vi "Mecanum_Calc.vi"(8 "Max Speed":dbl=3600.0, 11 "Drive Command Inputs":T1) -> (0 "error out":errorcluster, 3 "Drive Outputs":T2)   [LabVIEW 2012]
panel:
  in  "Dividing Factor":dbl=2.5
  in  "Set PID":bool
  in  "P Left":dbl
  in  "I Left":dbl=0.01
  in  "D Left":dbl
  in  "P Right":dbl
  in  "I Right":dbl=0.01
  in  "D Right":dbl
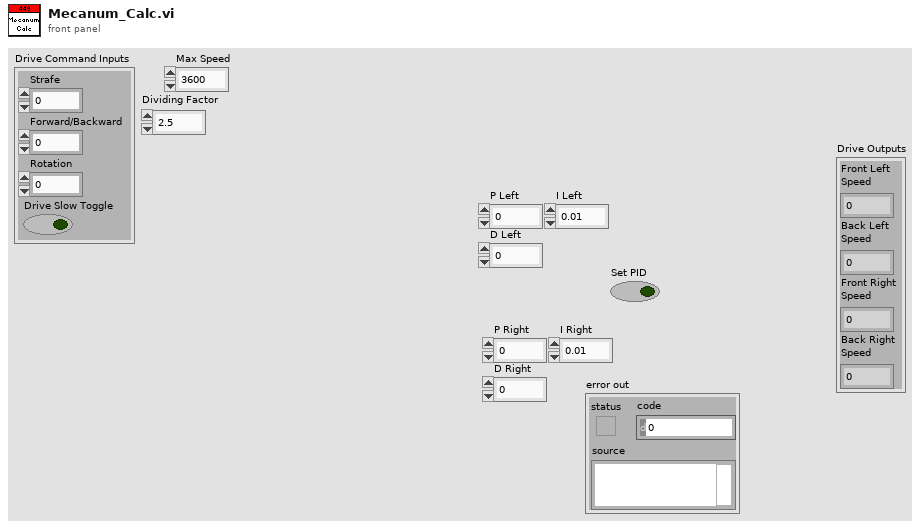
[diagram p1: front panel]
types:
  T1 = cluster{"Strafe":dbl, "Forward/Backward":dbl, "Rotation":dbl, "Drive Slow Toggle":bool}
  T2 = cluster{"Front Left\nSpeed":dbl, "Back Left\nSpeed":dbl, "Front Right\nSpeed":dbl, "Back Right\nSpeed":dbl}
  T3 = typedef "WPI_MotorControlDeviceRef.ctl" = cluster{"DeviceStatus":errorcluster, "Type":enum16{"PWM", "CAN"}, "PWM":cluster{"Digital Module":T4, "PWM Channel":T5, "DeadBand":T6}, "CAN":cluster{"Device Number":u8, "Control Mode":T7, "Semaphore":T8, "Max Vout":dbl}, "Invert":bool, "TransformRef":T9, "InvTransformRef":T9}
  T4 = typedef "FPGA_TypedefDigitalModule.ctl" = enum16{"Digital Module 1", "Digital Module 2"}
  T5 = typedef "FPGA_DIOPWMChannel.ctl" = enum8{"PWM 1", "PWM 2", "PWM 3", "PWM 4", "PWM 5", "PWM 6", "PWM 7", "PWM 8", "PWM 9", "PWM 10", "Invalid"}
  T6 = typedef "WPI_PWMDeadband.ctl" = cluster{"Name":string, "maxPositivePwm":i32, "minPositivePwm":i32, "centerPwm":i32, "maxNegativePwm":i32, "minNegativePwm":i32, "angularRange":u16}
  T7 = typedef "WPI_CANJaguar_ControlMode.ctl" = enum8{"Percent VBus", "Current", "Speed", "Position", "Voltage"}
  T8 = typedef "Semaphore RefNum" = refnum<k1>
  T9 = typedef "WPI_PWMTransform_ConPane.ctl" = refnum<vi>
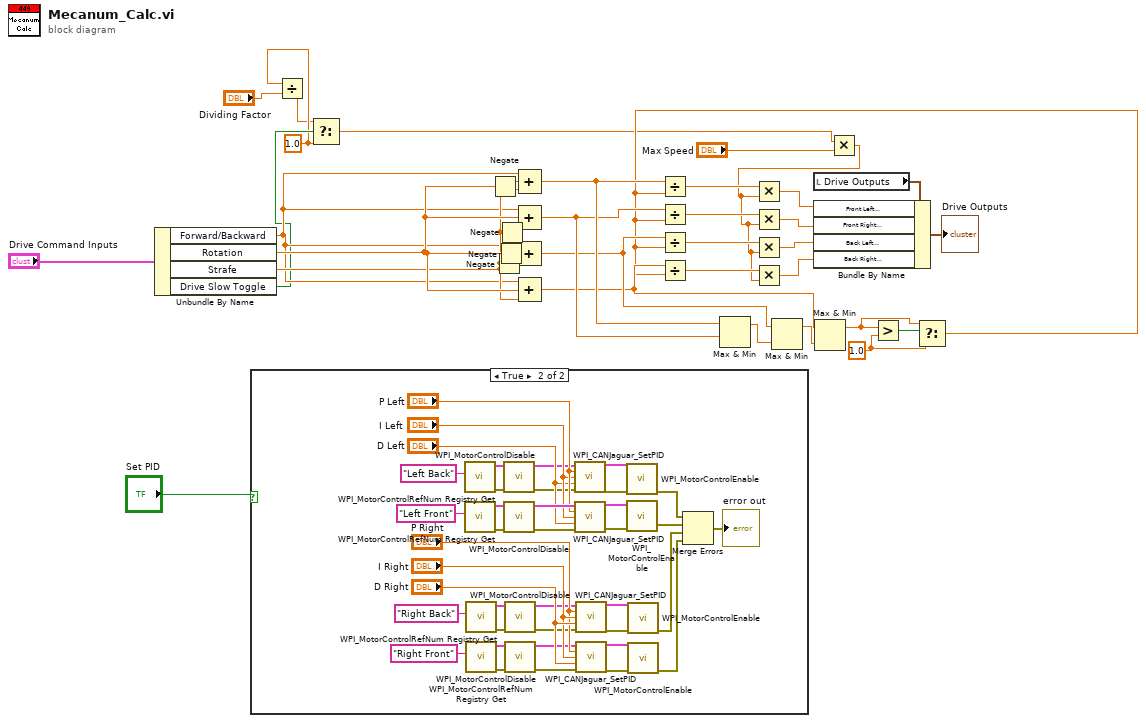
[diagram p0: block diagram]
diagram:
  w2 = 1.0 ("f")
  w17 = 1.0 ("y")
  n1 = Unbundle By Name("Drive Command Inputs") -> ("Forward/Backward"=w5:dbl, "Rotation"=w11:dbl, "Strafe"=w10:dbl, "Drive Slow Toggle"=w4:bool)
  n2 = case shown="True" "Set PID" {
    frame False {
    }
    frame True {
      n3 = call <vilib>:"WPI_MotorControlRefNum Registry Get.vi"("refnum name"="Left Back") -> ("error out"=w57:errorcluster, "MotorControlDevRef"=w56:T3)  [unwired: 9 in]
      n4 = call <vilib>:"WPI_MotorControlRefNum Registry Get.vi"("refnum name"="Left Front") -> ("error out"=w71:errorcluster, "MotorControlDevRef"=w72:T3)  [unwired: 9 in]
      n5 = call <vilib>:"WPI_MotorControlRefNum Registry Get.vi"("refnum name"="Right Back") -> ("error out"=w39:errorcluster, "MotorControlDevRef"=w40:T3)  [unwired: 9 in]
      n6 = call <vilib>:"WPI_MotorControlRefNum Registry Get.vi"("refnum name"="Right Front") -> ("error out"=w50:errorcluster, "MotorControlDevRef"=w49:T3)  [unwired: 9 in]
      n7 = call <vilib>:"WPI_MotorControlDisable.vi"("error in (no error)"=w57, "MotorControlDevRef"=w56) -> ("error out"=w54:errorcluster, "MotorControlDevRef"=w55:T3)  [unwired: 8 in]
      n8 = call <vilib>:"WPI_MotorControlDisable.vi"("error in (no error)"=w71, "MotorControlDevRef"=w72) -> ("error out"=w74:errorcluster, "MotorControlDevRef"=w73:T3)  [unwired: 8 in]
      n9 = call <vilib>:"WPI_MotorControlDisable.vi"("error in (no error)"=w39, "MotorControlDevRef"=w40) -> ("error out"=w42:errorcluster, "MotorControlDevRef"=w41:T3)  [unwired: 8 in]
      n10 = call <vilib>:"WPI_MotorControlDisable.vi"("error in (no error)"=w50, "MotorControlDevRef"=w49) -> ("error out"=w47:errorcluster, "MotorControlDevRef"=w48:T3)  [unwired: 8 in]
      n11 = call <vilib>:"WPI_CANJaguar_SetPID.vi"("CAN Jaguar Ref"=w55, "P"="P Left", "I"="I Left", "D"="D Left", "error in (no error)"=w54) -> ("CAN Jaguar Ref Out"=w53:T3, "error out"=w52:errorcluster)  [unwired: 9 in]
      n12 = call <vilib>:"WPI_CANJaguar_SetPID.vi"("CAN Jaguar Ref"=w73, "P"="P Left", "I"="I Left", "D"="D Left", "error in (no error)"=w74) -> ("CAN Jaguar Ref Out"=w75:T3, "error out"=w37:errorcluster)  [unwired: 9 in]
      n13 = call <vilib>:"WPI_CANJaguar_SetPID.vi"("CAN Jaguar Ref"=w41, "P"="P Right", "I"="I Right", "D"="D Right", "error in (no error)"=w42) -> ("CAN Jaguar Ref Out"=w43:T3, "error out"=w44:errorcluster)  [unwired: 9 in]
      n14 = call <vilib>:"WPI_CANJaguar_SetPID.vi"("CAN Jaguar Ref"=w48, "P"="P Right", "I"="I Right", "D"="D Right", "error in (no error)"=w47) -> ("CAN Jaguar Ref Out"=w46:T3, "error out"=w45:errorcluster)  [unwired: 9 in]
      n15 = call <vilib>:"WPI_MotorControlEnable.vi"("error in (no error)"=w52, "CAN Jaguar Ref"=w53) -> ("error out"=w69:errorcluster)  [unwired: 8 in, 1 out]
      n16 = call <vilib>:"WPI_MotorControlEnable.vi"("error in (no error)"=w37, "CAN Jaguar Ref"=w75) -> ("error out"=w68:errorcluster)  [unwired: 8 in, 1 out]
      n17 = call <vilib>:"WPI_MotorControlEnable.vi"("error in (no error)"=w44, "CAN Jaguar Ref"=w43) -> ("error out"=w67:errorcluster)  [unwired: 8 in, 1 out]
      n18 = call <vilib>:"WPI_MotorControlEnable.vi"("error in (no error)"=w45, "CAN Jaguar Ref"=w46) -> ("error out"=w66:errorcluster)  [unwired: 8 in, 1 out]
      n19 = Merge Errors(w69, w68, w67, w66) -> (→"error out":errorcluster)
    }
  }
  n20 = Divide(x=w2, y="Dividing Factor") -> (x/y=w1:dbl)
  n21 = Select(t=w1, s=w4, f=w2) -> (s? t:f=w14:dbl)
  n22 = Negate(x=w11) -> (-x=w6:dbl)
  n23 = Negate(x=w10) -> (-x=w8:dbl)
  n24 = Negate(x=w11) -> (-x=w9:dbl)
  n25 = Negate(x=w10) -> (-x=w7:dbl)
  n26 = Compound Arithmetic op=ADD(w5, w6, w10) -> (w25:dbl)
  n27 = Compound Arithmetic op=ADD(w5, w11, w7) -> (w24:dbl)
  n28 = Compound Arithmetic op=ADD(w5, w9, w8) -> (w23:dbl)
  n29 = Compound Arithmetic op=ADD(w5, w11, w10) -> (w21:dbl)
  n30 = Max & Min(x=w25, y=w24) -> (max(x,y)=w22:dbl)  [unwired: 1 out]
  n31 = Max & Min(x=w23, y=w22) -> (max(x,y)=w20:dbl)  [unwired: 1 out]
  n32 = local read "Drive Outputs"() -> (w35:T2)
  n33 = Max & Min(x=w21, y=w20) -> (max(x,y)=w18:dbl)  [unwired: 1 out]
  n34 = Multiply(x=w14, y="Max Speed") -> (x*y=w12:dbl)
  n35 = Greater?(x=w18, y=w17) -> (0:w19:bool)
  n36 = Select(t=w18, s=w19, f=w17) -> (s? t:f=w16:dbl)
  n37 = Divide(x=w25, y=w16) -> (x/y=w26:dbl)
  n38 = Divide(x=w24, y=w16) -> (x/y=w31:dbl)
  n39 = Divide(x=w23, y=w16) -> (x/y=w34:dbl)
  n40 = Divide(x=w21, y=w16) -> (x/y=w33:dbl)
  n41 = Multiply(x=w26, y=w12) -> (x*y=w30:dbl)
  n42 = Multiply(x=w31, y=w12) -> (x*y=w29:dbl)
  n43 = Multiply(x=w34, y=w12) -> (x*y=w27:dbl)
  n44 = Multiply(x=w33, y=w12) -> (x*y=w28:dbl)
  n45 = Bundle By Name(cluster=w35, "Front Left\nSpeed"=w30, "Front Right\nSpeed"=w29, "Back Left\nSpeed"=w27, "Back Right\nSpeed"=w28) -> (→"Drive Outputs":T2)
